vi "Xml_Save_To_File.vi"(7 "Custom Path":path, 8 "error in (no error)":errorcluster, 9 "Filename":string, 10 "EXPERT Path Selector":T7=enum."Resources", 11 "Variant":variant) -> (0 "error out":errorcluster)   [LabVIEW 2024]
uses:
  controls/EXPERT_Path_Selector.ctl
  controls/QMH_UI_Cluster.ctl
  controls/QMH_UI_References.ctl
  controls/QMH_UI_Report.ctl
  controls/QMH_UI_Command.ctl
  controls/QMH_ICR_Command.ctl
  controls/QMH_Status.ctl
  <vilib>/NI/GXML/GXML.lvlib
panel:
  in  "QMH UI Cluster":T1
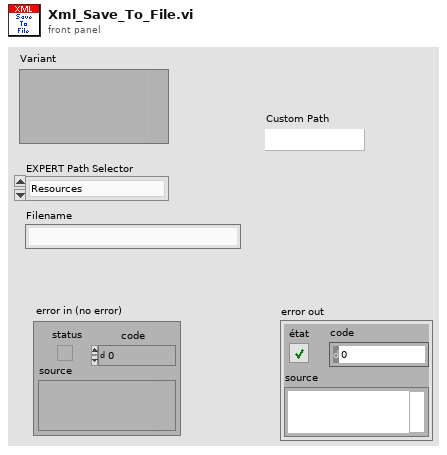
[diagram p1: front panel]
types:
  T1 = typedef "QMH_UI_Cluster.ctl" = cluster{"QMH UI References":T2, "QMH UI Report":T3}
  T2 = typedef "QMH_UI_References.ctl" = cluster{"Refnum Load":refnum<vi>, "Refnum Save As":refnum<vi>, "Refnum Start":refnum<vi>, "Refnum Exit":refnum<vi>, "Refnum Tabs":refnum<vi>, "Refnum SPECTRUM":refnum<vi>, "Refnum EXPERIMENT":refnum<vi>, "Refnum VOLTAGES":refnum<vi>, "Refnum SEQUENCE":refnum<vi>, "Refnum EXPERT":refnum<vi>, "Refnum LOOPS":refnum<vi>, "Refnum EXCIT Table":refnum<vi>, "Refnum TIMING Table":refnum<vi>, "Refnum CHANGE Experiment":refnum<vi>, "Refnum CHANGE Voltages":refnum<vi>, "Refnum CHANGE Sequence":refnum<vi>, "Refnum CHANGE Expert":refnum<vi>, "Refnum CHANGE Loops":refnum<vi>, "Refnum CHANGE Scientist":refnum<vi>, "Refnum PIL Status":refnum<vi>}
  T3 = typedef "QMH_UI_Report.ctl" = cluster{"UI Status":T4, "ICR Status":T5, "QMH Status":T6}
  T4 = typedef "QMH_UI_Command.ctl" = enum16{"Initialize", "UI Load", "UI Save", "UI Save As", "UI Change Experiment", "UI Change Voltages", "UI Change Sequence", "UI Change Expert", "UI Change Loops", "UI Change Scientist", "Ready to Start", "UI Start", "Waiting for ICR", "UI Exit", "Update Experiment", "Update Report", "Update ICR Status", "Waiting for User"}
  T5 = typedef "QMH_ICR_Command.ctl" = enum16{"Initialize", "Sequence Loop Setup", "Sequence Setup", "ICR Start", "ICR Stop", "Hardware Setup", "Next Sequence Loop", "Next Accumulation", "Waiting for Trigger", "Sequence Started", "Sequence Finished", "Sequence Loop Done", "Writing Data", "Hardware Reset", "Exit"}
  T6 = typedef "QMH_Status.ctl" = enum16{"Init", "Loading", "Setup", "Ready to Start", "Started", "Idle"}
  T7 = typedef "EXPERT_Path_Selector.ctl" = enum16{"Application", "Resources", "Data", "XML", "XML Saved", "Load Directory"}
  T8 = enum16{"open", "replace", "create", "open or create", "replace or create", "replace or create with confirmation"}
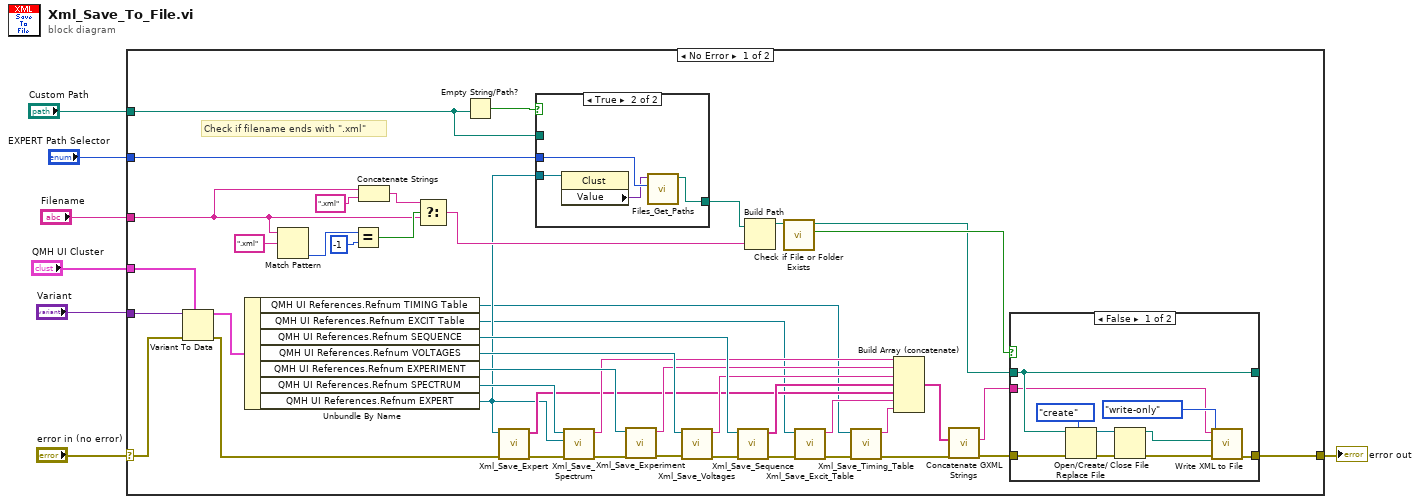
[diagram p0: block diagram]
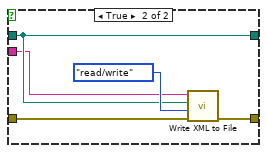
[diagram p3: hidden frame]
diagram:
  n1 = case shown="No Error" "error in (no error)" {
    selector: "error in (no error)" -> [w46 w73]
    tunnel: "Variant" -> [w29 _]
    tunnel: [w19 w73] -> w6
    tunnel: "Filename" -> [w23 _]
    tunnel: "EXPERT Path Selector" -> [w30 _]
    tunnel: "QMH UI Cluster" -> [w20 _]
    tunnel: "Custom Path" -> [w8 _]
    frame No Error {
      # "Check if filename ends with \".xml\""
      n2 = Variant To Data(error in=w46, type=w20, Variant=w29) -> (data=w45:T1, error out=w44:errorcluster)
      n3 = Unbundle By Name(w45) -> ("QMH UI References.Refnum TIMING Table"=w11:refnum<vi>, "QMH UI References.Refnum EXCIT Table"=w14:refnum<vi>, "QMH UI References.Refnum SEQUENCE"=w50:refnum<vi>, "QMH UI References.Refnum VOLTAGES"=w51:refnum<vi>, "QMH UI References.Refnum EXPERIMENT"=w52:refnum<vi>, "QMH UI References.Refnum SPECTRUM"=w47:refnum<vi>, "QMH UI References.Refnum EXPERT"=w16:refnum<vi>)
      n4 = Match Pattern(string=w23, regular expression=".xml" ("expression régulière")) -> (offset past match=w27:i32)  [unwired: 1 in, 3 out]
      n5 = Equal?(x=w27, y=-1) -> (x = y?=w25:bool)
      n6 = Concatenate Strings(w23, ".xml" ("chaîne")) -> (w24:string)
      n7 = Select(t=w24, s=w25, f=w23) -> (s? t:f=w21:string)
      n8 = Empty String/Path?(string/path=w8) -> (empty?=w9:bool)
      n9 = call "Xml_Save_Expert.vi"("error in (no error)"=w44, "Refnum Clust EXPERT"=w16) -> ("error out"=w18:errorcluster, "XML String Out"=w17:string[])  [unwired: 8 in]
      n10 = case shown="True" w9 {
        tunnel: [w53 w57] -> w31
        tunnel: w30 -> [_ w56]
        tunnel: w16 -> [_ w54]
        tunnel: w8 -> [w53 _]
        frame False {
        }
        frame True {
          n11 = property class="Clust"(reference=w54) -> ("Value"=w55:variant)  [unwired: 1 in, 2 out]
          n12 = call "Files_Get_Paths.vi"("EXPERT Path Selector"=w56, "Variant"=w55) -> ("Path"=w57:path)  [unwired: 8 in, 1 out]
        }
      }
      n13 = call "Xml_Save_Spectrum.vi"("error in (no error)"=w18, "Refnum Cluster\nEXPERT"=w16, "Refnum Cluster\nSPECTRUM"=w47) -> ("error out"=w48:errorcluster, "XML String Out"=w42:string)  [unwired: 7 in]
      n14 = call "Xml_Save_Experiment.vi"("error in (no error)"=w48, "Refnum Clust"=w52) -> ("error out"=w41:errorcluster, "XML String Out"=w38:string)  [unwired: 8 in]
      n15 = call "Xml_Save_Voltages.vi"("error in (no error)"=w41, "Refnum Clust"=w51) -> ("error out"=w40:errorcluster, "XML String Out"=w37:string)  [unwired: 8 in]
      n16 = call "Xml_Save_Sequence.vi"("error in (no error)"=w40, "Refnum Clust"=w50) -> ("error out"=w39:errorcluster, "XML String Out"=w43:string[])  [unwired: 8 in]
      n17 = Build Path(base path=w31, name or relative path=w21) -> (appended path=w36:path)
      n18 = call <vilib>:"Check if File or Folder Exists.vi"("path"=w36) -> ("file or folder exists?"=w35:bool, "dup path"=w34:path)  [unwired: 8 in, 1 out]
      n19 = call "Xml_Save_Excit_Table.vi"("error in (no error)"=w39, "Refnum Clust"=w14) -> ("error out"=w15:errorcluster, "XML String Out"=w13:string)  [unwired: 8 in]
      n20 = call "Xml_Save_Timing_Table.vi"("error in (no error)"=w15, "Refnum Clust"=w11) -> ("error out"=w12:errorcluster, "XML String Out"=w10:string)  [unwired: 8 in]
      n21 = Build Array (concatenate)(w42, w38, w37, w43, w17, w13, w10) -> (w49:string[])
      n22 = call <vilib>:"Concatenate GXML Strings.vi"("error in"=w12, "GXML Strings"=w49) -> ("error out"=w32:errorcluster, "Concatenated GXML String"=w33:string)  [unwired: 8 in]
      n23 = case shown="False" w35 {
        tunnel: w34 -> [w59 w69]
        tunnel: w33 -> [w58 w68]
        tunnel: w32 -> [w66 w71]
        tunnel: [w61 w70] -> w19
        tunnel: [w59 w69] -> _
        frame False {
          n24 = Open/Create/Replace File(file path (use dialog)=w59, error in=w66, operation (0:open)=T8."create" ("opération (0 : open)")) -> (refnum out=w63:refnum<file>, error out=w65:errorcluster)  [unwired: 3 in, 1 out]
          n25 = Close File(refnum=w63, error in=w65) -> (path=w60:path, error out=w64:errorcluster)
          n26 = call <vilib>:"Write XML to File.vi"("error in"=w64, "file access"=enum16{"read/write", "read-only", "write-only"}."write-only", "XML File Path"=w60, "XML Input"=w58) -> ("error out"=w61:errorcluster)  [unwired: 7 in]
        }
        frame True {
          n27 = call <vilib>:"Write XML to File.vi"("error in"=w71, "file access"=enum16{"read/write", "read-only", "write-only"}."read/write", "XML File Path"=w69, "XML Input"=w68) -> ("error out"=w70:errorcluster)  [unwired: 7 in]
        }
      }
    }
    frame Error {
    }
  }
  "error out" <- w6
